vi "Requests.vi"(8 "error in (no error)":errorcluster, 9 "write enable":bool=TRUE, 11 "ICPCON ET7042 in":refnum<class "ICPCON ET-7042UR.lvclass">) -> (0 "error out":errorcluster, 3 "ICPCON ET7042 out":refnum<class "ICPCON ET-7042UR.lvclass">)   [LabVIEW 2021, in "ICPCON ET-7042UR.lvclass"]
uses:
  ICPCON ET-7042UR.lvclass
  D:/my_projects/projects/Algorithms/Labview/21/Master CR/Master CR.lvclass
  D:/my_projects/projects/Algorithms/Labview/21/Master CR/Devices/ET7000/TCP/TCP.lvclass
  Master CR.lvclass/Master CR.ctl
  Modbus_v121c/Modbus Data Unit/Modbus Data Unit.lvclass/Modbus Data Unit.ctl
  Modbus_v121c/Network Protocol/Network Master/Network Master.lvclass/Network Master.ctl
  Network Protocol/Read Network Protocol.vi
  Modbus_v121c/Master Function Definition/Read Coils Request.vi
  Modbus_v121c/Network Protocol/Network Master/Read write Master.vi
  Modbus_v121c/Master Function Definition/Read Coils Response.vi
  Modbus_v121c/Master Function Definition/Write Multiple Coils Request.vi
  Modbus_v121c/Master Function Definition/Function data mismatch error.vi
  Modbus_v121c/Master Function Definition/Write Multiple Coils Response.vi
  Modbus_v121c/Modbus Data Unit/Construct PDU.vi
  Modbus_v121c/Utility/Bytes to Bits.vi
  Modbus_v121c/Data Model/Error Generator.vi
  Modbus_v121c/Master Function Definition/Function code mismatch error.vi
  Modbus_v121c/Modbus Data Unit/Deconstruct PDU.vi
  Modbus_v121c/Utility/Bits to Bytes.vi
  TCP/TCP.lvclass
  Modbus_v121c/Network Protocol/Network Master/Network Master.lvclass
  Modbus_v121c/Modbus Data Unit/Modbus Data Unit.lvclass
  Modbus_v121c/Data Model/Device Data Model.lvclass
  Modbus_v121c/Transmission Data Unit/Transmission Data Unit.lvclass
  Master CR.lvclass
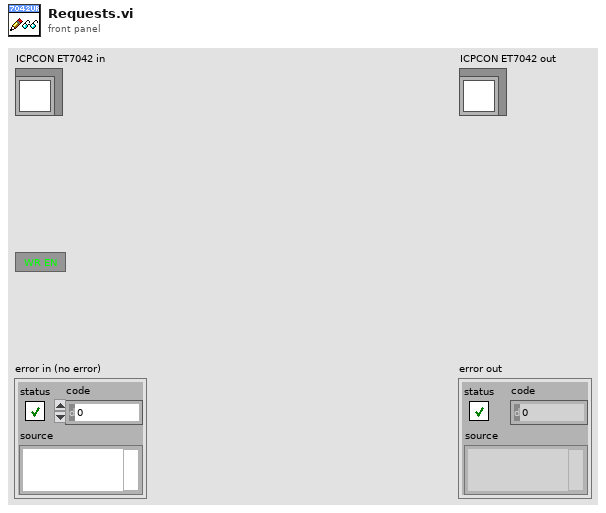
[diagram p1: front panel]
types:
  T1 = typedef "Device Data Model.lvclass/N channel.ctl" = cluster{"N DI channel":i32, "N DO channel":i32, "N AI channel":i32, "N AO channel":i32}
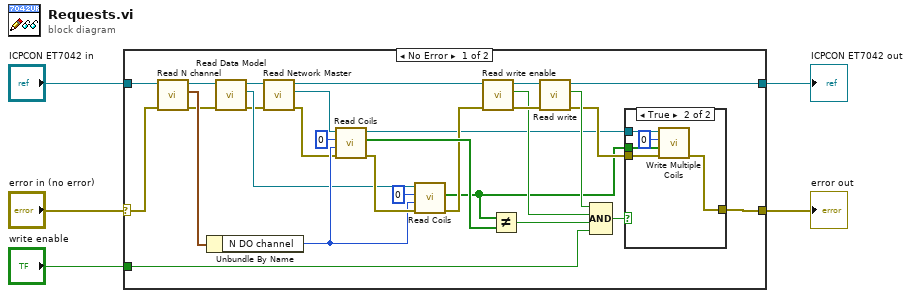
[diagram p0: block diagram]
diagram:
  n1 = case shown="No Error" "error in (no error)" {
    selector: "error in (no error)" -> [w31 w42]
    tunnel: [w17 w42] -> w3
    tunnel: [w6 w41] -> w4
    tunnel: "ICPCON ET7042 in" -> [w33 w41]
    tunnel: "write enable" -> [w18 _]
    frame No Error {
      n2 = call "Read N channel.vi"("error in (no error)"=w31, "Master CR in"=w33) -> ("error out"=w30:errorcluster, "N channel"=w34:T1, "Master CR out"=w32:refnum<class "ICPCON ET-7042UR.lvclass">)  [unwired: 7 in]
      n3 = Unbundle By Name(w34) -> ("N DO channel"=w20:i32)
      n4 = call "Read Data Model.vi"("error in (no error)"=w30, "Master CR in"=w32) -> ("error out"=w11:errorcluster, "Data Model"=w16:refnum<class "Device Data Model.lvclass">, "Master CR out"=w12:refnum<class "ICPCON ET-7042UR.lvclass">)  [unwired: 7 in]
      n5 = call "Read Network Master.vi"("error in (no error)"=w11, "TCP in"=w12) -> ("error out"=w10:errorcluster, "Network Master"=w8:refnum<class "Network Master.lvclass">, "TCP out"=w9:refnum<class "ICPCON ET-7042UR.lvclass">)  [unwired: 7 in]
      n6 = call "Read Coils.vi"("error in (no error)"=w10, "number of coils"=w20, "starting address"=u16 0, "Modbus master in"=w8) -> ("error out"=w22:errorcluster, "coil values"=w23:bool[], "Modbus master out"=w7:refnum<class "Network Master.lvclass">)  [unwired: 5 in]
      n7 = call-dynamic "Read Coils.vi"("error in"=w22, "number of coils"=w20, "starting address"=u16 0, "device data model in"=w16) -> ("error out"=w15:errorcluster, "data"=w13:bool[])  [unwired: 5 in, 1 out]
      n8 = call "Read write enable.vi"("error in (no error)"=w15, "Master CR in"=w9) -> ("error out"=w28:errorcluster, "write enable"=w24:bool, "Master CR out"=w29:refnum<class "ICPCON ET-7042UR.lvclass">)  [unwired: 7 in]
      n9 = Not Equal?(x=w13, y=w23) -> (x != y?=w27:bool)
      n10 = call "Read write.vi"("error in (no error)"=w28, "Master CR in"=w29) -> ("error out"=w14:errorcluster, "Write"=w25:bool, "Master CR out"=w6:refnum<class "ICPCON ET-7042UR.lvclass">)  [unwired: 7 in]
      n11 = Compound Arithmetic op=AND(w25, w24, w27, w18) -> (w26:bool)
      n12 = case shown="True" w26 {
        tunnel: w14 -> [w35 w40]
        tunnel: [w35 w37] -> w17
        tunnel: w13 -> [_ w39]
        tunnel: w7 -> [_ w36]
        frame False {
        }
        frame True {
          n13 = call "Write Multiple Coils.vi"("error in (no error)"=w40, "coil values"=w39, "starting address"=u16 0, "Modbus master in"=w36) -> ("error out"=w37:errorcluster)  [unwired: 6 in, 1 out]
        }
      }
    }
    frame Error {
    }
  }
  "error out" <- w3
  "ICPCON ET7042 out" <- w4
